vi "DAQmx_SwitchLineDirection.vi"() -> ()   [LabVIEW 2020]
uses:
  <vilib>/DAQmx/write.llb/DAQmx Write (Digital Bool 1Line 1Point).vi
  <vilib>/DAQmx/read.llb/DAQmx Read (Digital Bool 1Line 1Point).vi
  <vilib>/DAQmx/miscellaneous.llb/DAQmx Fill In Error Info.vi
panel:
  out "error out":errorcluster
  in  "error in (no error)":errorcluster
  in  "DO.Line":tag="NI-USB6509/port0/line0" caption="Line"
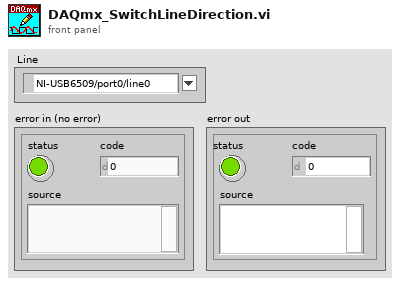
[diagram p1: front panel]
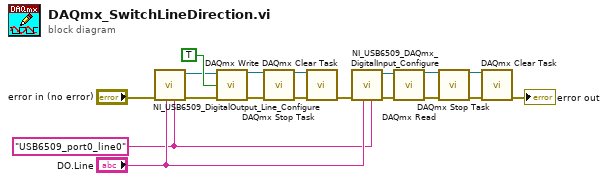
[diagram p0: block diagram]
diagram:
  w1 = "USB6509_port0_line0" ("TasklName")
  n1 = call "NI_USB6509_DigitalOutput_Line_Configure.vi"("TasklName"=w1, "DO.Line"="DO.Line", "error in (no error)"="error in (no error)") -> ("error out"=w17:errorcluster, "DAQmx.DO.Tast"=w11:refnum<k21>)  [unwired: 7 in]
  n2 = call-poly <vilib>:"DAQmx Write.vi"("task/channels in"=w11, "data"=TRUE, "error in"=w17) -> ("task out"=w13:refnum<k21>, "error out"=w14:errorcluster)  [unwired: 10 in, 1 out]
  n3 = call <vilib>:"DAQmx Stop Task.vi"("task/channels in"=w13, "error in"=w14) -> ("task out"=w12:refnum<k21>, "error out"=w15:errorcluster)  [unwired: 12 in]
  n4 = call <vilib>:"DAQmx Clear Task.vi"("task in"=w12, "error in"=w15) -> ("error out"=w3:errorcluster)  [unwired: 13 in]
  n5 = call "NI_USB6509_DAQmx_DigitalInput_Configure.vi"("TasklName"=w1, "DO.Line"="DO.Line", "error in (no error)"=w3) -> ("error out"=w5:errorcluster, "Refnum out"=w4:refnum<k21>)  [unwired: 7 in]
  n6 = call-poly <vilib>:"DAQmx Read.vi"("task/channels in"=w4, "error in"=w5) -> ("task out"=w6:refnum<k21>, "error out"=w8:errorcluster)  [unwired: 11 in, 1 out]
  n7 = call <vilib>:"DAQmx Stop Task.vi"("task/channels in"=w6, "error in"=w8) -> ("task out"=w10:refnum<k21>, "error out"=w9:errorcluster)  [unwired: 12 in]
  n8 = call <vilib>:"DAQmx Clear Task.vi"("task in"=w10, "error in"=w9) -> ("error out"=→"error out":errorcluster)  [unwired: 13 in]
